vi "Kicker and Roller Control.vi"() -> ()   [LabVIEW 2011]
uses:
  <vilib>/Rock Robotics/WPI/Solenoid/WPI_SolenoidValue.ctl
  <vilib>/Rock Robotics/WPI/Solenoid/WPI_SolenoidSetEnum.vi
panel:
  in  "Delay (ms)":u32=500
  in  "chambering speed":dbl=0.55
  in  "intake speed":dbl=1.0
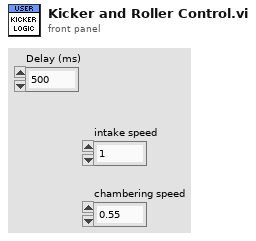
[diagram p1: front panel]
types:
  T1 = enum16{"Intake", "Chambering Front", "Chambering Rear"}
  T2 = typedef "WPI_JoystickDevRef.ctl" = cluster{"Device":T3}
  T3 = typedef "WPI_JoystickDeviceEnum.ctl" = enum16{"USB 1", "USB 2", "USB 3", "USB 4", "Kinect 1", "Kinect 2"}
  T4 = typedef "WPI_JoystickButtonState.ctl" = cluster{"Button 1":bool, "Button 2":bool, "Button 3":bool, "Button 4":bool, "Button 5":bool, "Button 6":bool, "Button 7":bool, "Button 8":bool, "Button 9":bool, "Button 10":bool, "Button 11":bool, "Button 12":bool}
  T5 = typedef "WPI_DigitalInputDevRef.ctl" = cluster{"DevStatus":errorcluster, "DIO Channel":T6, "Digital Module":T7}
  T6 = typedef "FPGA_DIOChannel.ctl" = enum8{"DIO 1", "DIO 2", "DIO 3", "DIO 4", "DIO 5", "DIO 6", "DIO 7", "DIO 8", "DIO 9", "DIO 10", "DIO 11", "DIO 12", "DIO 13", "DIO 14", "Invalid"}
  T7 = typedef "FPGA_TypedefDigitalModule.ctl" = enum16{"Digital Module 1", "Digital Module 2"}
  T8 = typedef "WPI_SolenoidDevRef.ctl" = cluster{"DevStatus":errorcluster, "Solenoid Module":T9, "Forward Solenoid Channel":T10, "Reverse Solenoid Channel":T10}
  T9 = typedef "FPGA_TypedefSolenoidModule.ctl" = enum16{"Solenoid Module 1", "Solenoid Module 2"}
  T10 = typedef "WPI_SolenoidChannel.ctl" = enum8{"Solenoid 1", "Solenoid 2", "Solenoid 3", "Solenoid 4", "Solenoid 5", "Solenoid 6", "Solenoid 7", "Solenoid 8", "Invalid"}
  T11 = typedef "WPI_MotorControlDeviceRef.ctl" = cluster{"DeviceStatus":errorcluster, "Type":enum16{"PWM", "CAN"}, "PWM":cluster{"Digital Module":T7, "PWM Channel":T12, "DeadBand":T13}, "CAN":cluster{"Device Number":u8, "Control Mode":T14, "Semaphore":T15, "Max Vout":dbl}, "Invert":bool, "TransformRef":T16, "InvTransformRef":T16}
  T12 = typedef "FPGA_DIOPWMChannel.ctl" = enum8{"PWM 1", "PWM 2", "PWM 3", "PWM 4", "PWM 5", "PWM 6", "PWM 7", "PWM 8", "PWM 9", "PWM 10", "Invalid"}
  T13 = typedef "WPI_PWMDeadband.ctl" = cluster{"Name":string, "maxPositivePwm":i32, "minPositivePwm":i32, "centerPwm":i32, "maxNegativePwm":i32, "minNegativePwm":i32, "angularRange":u16}
  T14 = typedef "WPI_CANJaguar_ControlMode.ctl" = enum8{"Percent VBus", "Current", "Speed", "Position", "Voltage"}
  T15 = typedef "Semaphore RefNum" = refnum<k1>
  T16 = typedef "WPI_PWMTransform_ConPane.ctl" = refnum<vi>
  T17 = typedef "WPI_SolenoidValue.ctl" = enum16{"Off", "On", "Forward", "Reverse"}
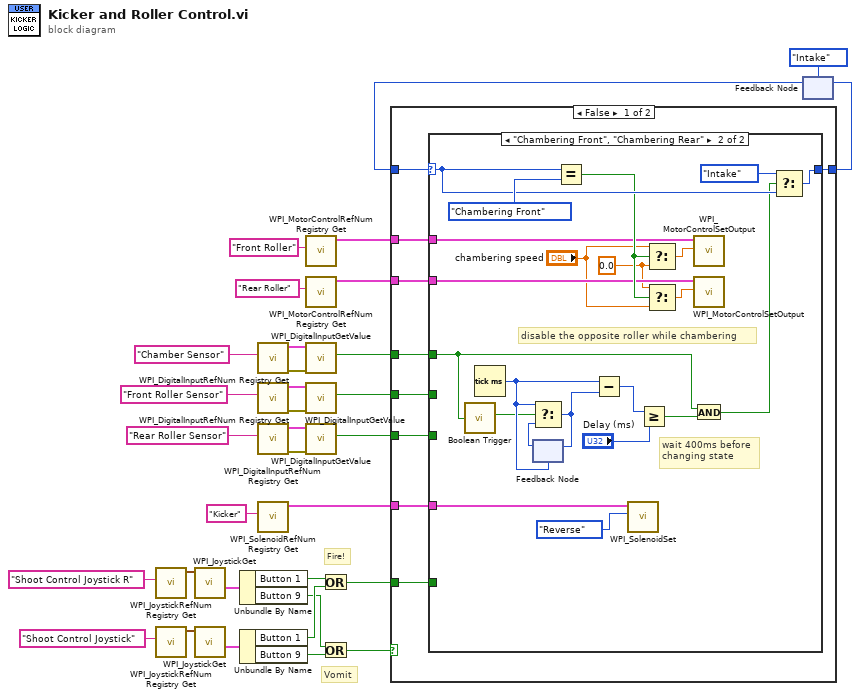
[diagram p0: block diagram]
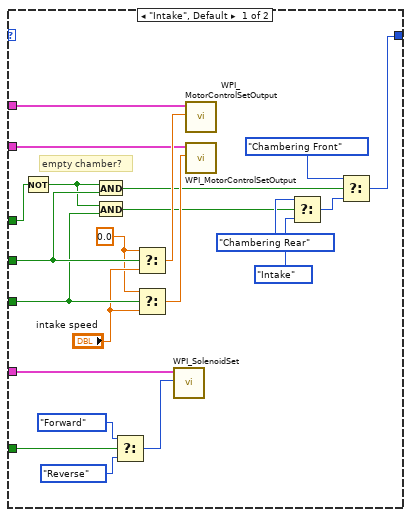
[diagram p2: hidden frame]
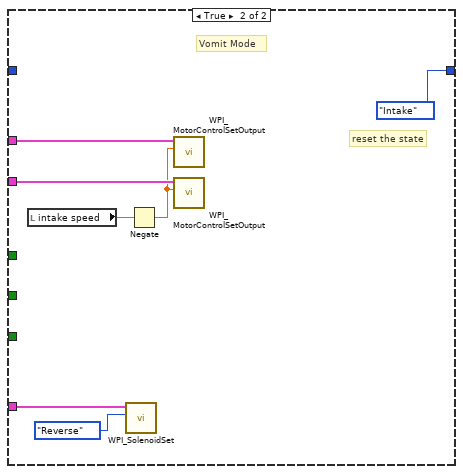
[diagram p3: hidden frame]
diagram:
  # "Vomit"
  # "Fire!"
  n1 = call <vilib>:"WPI_JoystickRefNum Registry Get.vi"("refnum name"="Shoot Control Joystick R") -> ("JoystickDevRef"=w20:T2)  [unwired: 9 in, 1 out]
  n2 = call <vilib>:"WPI_JoystickRefNum Registry Get.vi"("refnum name"="Shoot Control Joystick") -> ("JoystickDevRef"=w23:T2)  [unwired: 9 in, 1 out]
  n3 = call <vilib>:"WPI_JoystickGet.vi"("JoystickDevRef"=w20) -> ("Buttons"=w19:T4)  [unwired: 4 in, 2 out]
  n4 = call <vilib>:"WPI_JoystickGet.vi"("JoystickDevRef"=w23) -> ("Buttons"=w22:T4)  [unwired: 4 in, 2 out]
  n5 = Unbundle By Name(w19) -> ("Button 1"=w18:bool, "Button 9"=w13:bool)
  n6 = Unbundle By Name(w22) -> ("Button 1"=w17:bool, "Button 9"=w14:bool)
  n7 = call <vilib>:"WPI_DigitalInputRefNum Registry Get.vi"("refnum name"="Chamber Sensor") -> ("error out"=w31:errorcluster, "DigitalInputDevRef"=w32:T5)  [unwired: 9 in]
  n8 = call <vilib>:"WPI_DigitalInputRefNum Registry Get.vi"("refnum name"="Front Roller Sensor") -> ("error out"=w30:errorcluster, "DigitalInputDevRef"=w29:T5)  [unwired: 9 in]
  n9 = call <vilib>:"WPI_DigitalInputRefNum Registry Get.vi"("refnum name"="Rear Roller Sensor") -> ("error out"=w25:errorcluster, "DigitalInputDevRef"=w26:T5)  [unwired: 9 in]
  n10 = call <vilib>:"WPI_SolenoidRefNum Registry Get.vi"("refnum name"="Kicker") -> ("SolenoidDevRef"=w2:T8)  [unwired: 9 in, 1 out]
  n11 = call <vilib>:"WPI_MotorControlRefNum Registry Get.vi"("refnum name"="Front Roller") -> ("MotorControlDevRef"=w10:T11)  [unwired: 9 in, 1 out]
  n12 = call <vilib>:"WPI_MotorControlRefNum Registry Get.vi"("refnum name"="Rear Roller") -> ("MotorControlDevRef"=w9:T11)  [unwired: 9 in, 1 out]
  n13 = call <vilib>:"WPI_DigitalInputGetValue.vi"("error in (no error)"=w31, "DigitalInputDevRef"=w32) -> ("Value"=w3:bool)  [unwired: 7 in, 2 out]
  n14 = call <vilib>:"WPI_DigitalInputGetValue.vi"("error in (no error)"=w30, "DigitalInputDevRef"=w29) -> ("Value"=w5:bool)  [unwired: 7 in, 2 out]
  n15 = call <vilib>:"WPI_DigitalInputGetValue.vi"("error in (no error)"=w25, "DigitalInputDevRef"=w26) -> ("Value"=w4:bool)  [unwired: 7 in, 2 out]
  n16 = Or(x=w18, y=w17) -> (x .or. y?=w1:bool)
  n17 = Or(x=w13, y=w14) -> (x .or. y?=w12:bool)
  n18 = feedback #1(T1."Intake") -> (w8:T1)
  n19 = case shown="False" w12 {
    tunnel: w10 -> [w40 w90]
    tunnel: w9 -> [w38 w89]
    tunnel: w8 -> [w42 _]
    tunnel: [w37 T1."Intake"] -> w7
    tunnel: w5 -> [w41 _]
    tunnel: w4 -> [w39 _]
    tunnel: w3 -> [w36 _]
    tunnel: w2 -> [w35 w92]
    tunnel: w1 -> [w34 _]
    frame False {
      n20 = case shown="\"Chambering Front\", \"Chambering Rear\"" w42 {
        selector: w42 -> [_ w85]
        tunnel: w41 -> [w56 _]
        tunnel: w40 -> [w46 w76]
        tunnel: w39 -> [w53 _]
        tunnel: w38 -> [w45 w77]
        tunnel: [w62 w84] -> w37
        tunnel: w36 -> [w57 w67]
        tunnel: w35 -> [w51 w78]
        tunnel: w34 -> [w50 _]
        frame "Intake", Default {
          w43 = 0.0 ("t")
          # "empty chamber?"
          n21 = Not(x=w57) -> (.not. x?=w52:bool)
          n22 = And(x=w52, y=w56) -> (x .and. y?=w55:bool)
          n23 = And(x=w52, y=w53) -> (x .and. y?=w54:bool)
          n24 = Select(t=WPI_SolenoidValue."Forward", s=w50, f=WPI_SolenoidValue."Reverse" ("Value")) -> (s? t:f=w48:T17)
          n25 = Select(t=w43, s=w56, f="intake speed") -> (s? t:f=w64:dbl)
          n26 = Select(t=w43, s=w53, f="intake speed") -> (s? t:f=w63:dbl)
          n27 = call-poly <vilib>:"WPI_SolenoidSet.vi"("Value"=w48, "SolenoidDevRef"=w51) -> ()  [unwired: 8 in, 2 out]
          n28 = call <vilib>:"WPI_MotorControlSetOutput.vi"("Output"=w64, "MotorControlDevRef"=w46) -> ()  [unwired: 8 in, 2 out]
          n29 = call <vilib>:"WPI_MotorControlSetOutput.vi"("Output"=w63, "MotorControlDevRef"=w45) -> ()  [unwired: 8 in, 2 out]
          n30 = Select(t=T1."Chambering Rear", s=w54, f=T1."Intake") -> (s? t:f=w60:T1)
          n31 = Select(t=T1."Chambering Front", s=w55, f=w60) -> (s? t:f=w62:T1)
        }
        frame "Chambering Front", "Chambering Rear" {
          w74 = 0.0 ("f")
          # "wait 400ms before\nchanging state"
          # "disable the opposite roller while chambering"
          n32 = call "Boolean Trigger.vi"("input"=w67) -> ("rising edge"=w68:bool)  [unwired: 2 in, 1 out]
          n33 = Tick Count (ms)() -> (millisecond timer value=w70:u32)
          n34 = feedback #2(w70) -> (w69:u32)
          n35 = Select(t=w70, s=w68, f=w69) -> (s? t:f=w71:u32)
          n36 = feedback-in #2(w71) -> ()
          n37 = Equal?(x=w85, y=T1."Chambering Front") -> (x = y?=w80:bool)
          n38 = Subtract(x=w70, y=w71) -> (x-y=w72:u32)
          n39 = call-poly <vilib>:"WPI_SolenoidSet.vi"("Value"=WPI_SolenoidValue."Reverse", "SolenoidDevRef"=w78) -> ()  [unwired: 8 in, 2 out]
          n40 = Greater Or Equal?(x=w72, y="Delay (ms)") -> (x >= y?=w73:bool)
          n41 = Select(t="chambering speed", s=w80, f=w74) -> (s? t:f=w82:dbl)
          n42 = Select(t=w74, s=w80, f="chambering speed") -> (s? t:f=w81:dbl)
          n43 = call <vilib>:"WPI_MotorControlSetOutput.vi"("Output"=w82, "MotorControlDevRef"=w76) -> ()  [unwired: 8 in, 2 out]
          n44 = call <vilib>:"WPI_MotorControlSetOutput.vi"("Output"=w81, "MotorControlDevRef"=w77) -> ()  [unwired: 8 in, 2 out]
          n45 = And(x=w67, y=w73) -> (x .and. y?=w66:bool)
          n46 = Select(t=T1."Intake", s=w66, f=w85) -> (s? t:f=w84:T1)
        }
      }
    }
    frame True {
      # "Vomit Mode"
      # "reset the state"
      n47 = local read "intake speed"() -> (w88:dbl)
      n48 = call-poly <vilib>:"WPI_SolenoidSet.vi"("Value"=WPI_SolenoidValue."Reverse", "SolenoidDevRef"=w92) -> ()  [unwired: 8 in, 2 out]
      n49 = Negate(x=w88) -> (-x=w87:dbl)
      n50 = call <vilib>:"WPI_MotorControlSetOutput.vi"("Output"=w87, "MotorControlDevRef"=w90) -> ()  [unwired: 8 in, 2 out]
      n51 = call <vilib>:"WPI_MotorControlSetOutput.vi"("Output"=w87, "MotorControlDevRef"=w89) -> ()  [unwired: 8 in, 2 out]
    }
  }
  n52 = feedback-in #1(w7) -> ()
